vi "position_loader.vi"() -> ()   [LabVIEW 2016]
panel:
  out "element":dbl
  in  "disabled index (col)":i32
  in  "index (row)":i32
  out "array":dbl[][](array[numeric])
  out "text":string
  in  "File Path Control":path
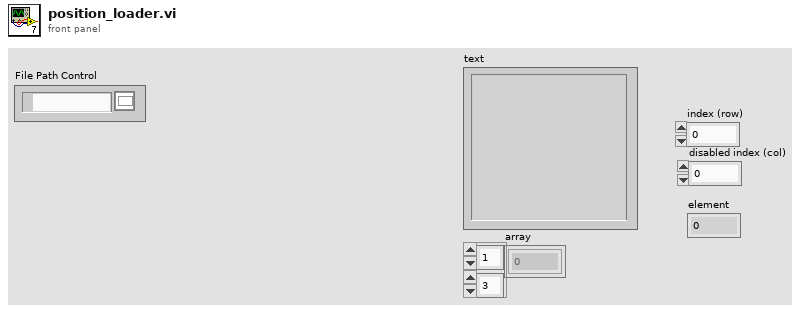
[diagram p1: front panel]
types:
  T1 = enum16{"open", "replace", "create", "open or create", "replace or create", "replace or create with confirmation"}
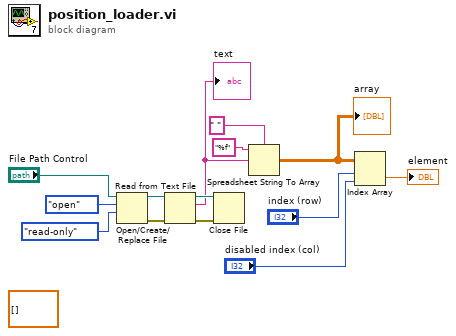
[diagram p0: block diagram]
diagram:
  (unwired) dbl[][] [] ("array type (2D Dbl)")
  n1 = Open/Create/Replace File(file path (use dialog)="File Path Control", operation (0:open)=T1."open", access (0:read/write)=enum16{"read/write", "read-only", "write-only"}."read-only") -> (refnum out=w11:refnum<file>, error out=w8:errorcluster)  [unwired: 3 in, 1 out]
  n2 = Read from Text File(file (use dialog)=w11, error in=w8) -> (refnum out=w10:refnum<file>, text=w7:string, error out=w9:errorcluster)  [unwired: 2 in, 1 out]
  "text" <- w7
  n3 = Close File(refnum=w10, error in=w9) -> ()  [unwired: 2 out]
  n4 = Spreadsheet String To Array(delimiter (Tab)=" ", format string="%f", spreadsheet string=w7) -> (array=w4:dbl[][])  [unwired: 1 in]
  "array" <- w4
  n5 = Index Array(array=w4, index (row)="index (row)", index (col)="disabled index (col)") -> (element=→"element":dbl)
